vi "Parse Session (Rx-Monitor).vi"(8 "error in":errorcluster, 11 "node in":refnum<k20>) -> (0 "error out":errorcluster, 3 "session_rx_monitor":T1={"DefaultCronoMode"=1, "GlbMonBufferSizeIn"=0, "CaptureMode"=0, "MaxFileSizeMB"=1, "Strobe"=0, "TriggerPosition"=0} {"Strobe" items=["FDX_MON_STROBE_DIS", "FDX_MON_STROBE_STOP", "FDX_MON_STROBE_START"]; "CaptureMode" items=["FDX_MON_SINGLE ", "FDX_MON_CONTINUOUS", "FDX_MON_SELECTIVE", "FDX_MON_RECORDING", "FDX_MON_REROS", "FDX_MON_HMU"]; "DefaultCronoMode" items=["FDX_RX_DEFAULT_ENA_CNT", "FDX_RX_DEFAULT_MON_ENA_ALL", "FDX_RX_DEFAULT_MON_ENA_GOOD"]})   [LabVIEW 2020, in "AIM ARINC 664 Import.lvlib"]
uses:
  AIM ARINC 664 Import.lvlib
  _typedefs/session_rx_monitor.ctl
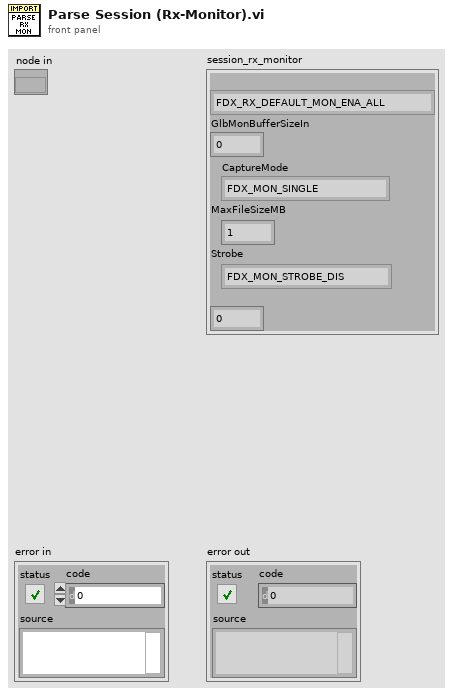
[diagram p1: front panel]
types:
  T1 = typedef "AIM ARINC 664 Import.lvlib/session_rx_monitor.ctl" = cluster{"DefaultCronoMode":u32, "GlbMonBufferSizeIn":u32, "CaptureMode":u32, "MaxFileSizeMB":u32, "Strobe":u32, "TriggerPosition":u32}
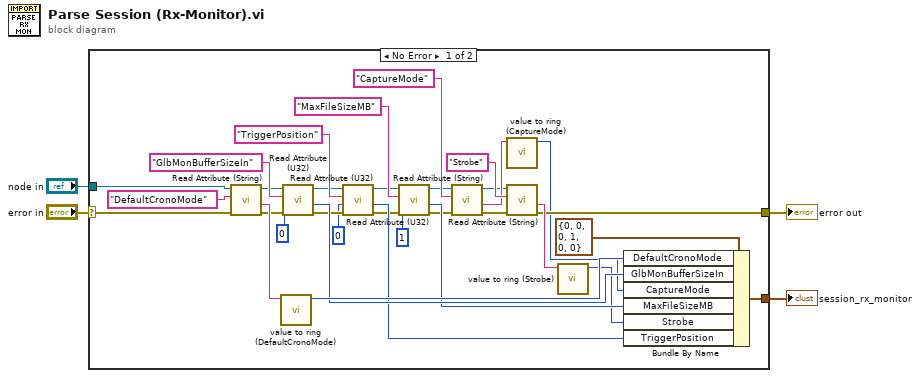
[diagram p0: block diagram]
diagram:
  n1 = case shown="No Error" "error in" {
    selector: "error in" -> [w36 w38]
    tunnel: "node in" -> [w37 _]
    tunnel: [w10 w38] -> w3
    tunnel: [w33 _] -> w1
    frame No Error {
      n2 = call "Read Attribute (String).vi"("error in"=w36, "Attribute Name"="DefaultCronoMode" ("Tag Name"), "node in"=w37) -> ("error out"=w25:errorcluster, "value"=w32:string, "node out"=w24:refnum<k20>)  [unwired: 6 in]
      n3 = call "value to ring (DefaultCronoMode).vi"("value"=w32) -> ("DefaultCronoMode"=w31:u32)  [unwired: 10 in]
      n4 = call "Read Attribute (U32).vi"("error in"=w25, "default"=u32 0, "Attribute Name"="GlbMonBufferSizeIn" ("Tag Name"), "node in"=w24) -> ("error out"=w22:errorcluster, "value"=w23:u32, "node out"=w18:refnum<k20>)  [unwired: 5 in]
      n5 = call "Read Attribute (U32).vi"("error in"=w22, "default"=u32 0, "Attribute Name"="TriggerPosition" ("Tag Name"), "node in"=w18) -> ("error out"=w19:errorcluster, "value"=w21:u32, "node out"=w17:refnum<k20>)  [unwired: 5 in]
      n6 = call "Read Attribute (U32).vi"("error in"=w19, "default"=u32 1, "Attribute Name"="MaxFileSizeMB" ("Tag Name"), "node in"=w17) -> ("error out"=w16:errorcluster, "value"=w20:u32, "node out"=w15:refnum<k20>)  [unwired: 5 in]
      n7 = call "Read Attribute (String).vi"("error in"=w16, "Attribute Name"="CaptureMode" ("Tag Name"), "node in"=w15) -> ("error out"=w11:errorcluster, "value"=w14:string, "node out"=w12:refnum<k20>)  [unwired: 6 in]
      n8 = call "value to ring (CaptureMode).vi"("value"=w14) -> ("CaptureMode"=w9:u32)  [unwired: 10 in]
      n9 = call "Read Attribute (String).vi"("error in"=w11, "Attribute Name"="Strobe" ("Tag Name"), "node in"=w12) -> ("error out"=w10:errorcluster, "value"=w13:string)  [unwired: 6 in, 1 out]
      n10 = call "value to ring (Strobe).vi"("value"=w13) -> ("Strobe"=w8:u32)  [unwired: 10 in]
      n11 = Bundle By Name(cluster=T1 {"DefaultCronoMode"=0, "GlbMonBufferSizeIn"=0, "CaptureMode"=0, "MaxFileSizeMB"=1, "Strobe"=0, "TriggerPosition"=0} ("session_rx_monitor"), "DefaultCronoMode"=w31, "GlbMonBufferSizeIn"=w23, "CaptureMode"=w9, "MaxFileSizeMB"=w20, "Strobe"=w8, "TriggerPosition"=w21) -> (w33:T1)
    }
    frame Error {
    }
  }
  "error out" <- w3
  "session_rx_monitor" <- w1
